vi "Group Terminals.vi"(6 "State":T8={"Worker Library Path"=path "", "Block Label"="", "Types"=[], "Selections"=[], "Icon"={"image type"=0, "image depth"=0, "image"=[], "mask"=[], "colors"=[], "Rectangle"={"left"=0, "top"=0, "right"=0, "bottom"=0}}, "Errors"={"Terminals"=[], "Generate"={"status"=FALSE, "code"=0, "source"=""}, "General"={"status"=FALSE, "code"=0, "source"=""}}, "Calculated Sizes"={"Block Width"=0, "Block Height"=0, "Half Width"=0, "Icon Top"=0, "Icon Bottom"=0, "Label Width"=0, "Half Label"=0, "Label Top"=0, "Text Width"=0, "Half Text"=0, "Text Height"=0, "Label Height"=0, "Expanded Width"=0, "Label Bottom"=0, "Expanded Top"=0, "Expanded Bottom"=0, "Expanded Height"=0, "Min Height"=0, "Max Height"=0}, "Special Terminal Indices"={"Action"=-1, "Init"=-1, "Tag"=-1, "State in"=-1, "State out"=-1, "Error"=-1}, "Terminals"=[]}, 8 "error in (no error)":errorcluster, 11 "Refs In":T15) -> (0 "error out":errorcluster, 2 "Grouped Terms":T1, 3 "Refs":T15)   [LabVIEW 2022 SP3, in "FlexBlocks Support.lvlib"]
uses:
  FlexBlocks Support.lvlib
  SM Refs.ctl
  Flex Block/State.ctl
  Type Descriptor.ctl
  Terminal Direction.ctl
  Value Mode.ctl
  Special Terminal.ctl
  <vilib>/picture/picture.llb/imagedata.ctl
  XNode Errors.ctl
  Calculated Sizes.ctl
  Special Terminal Indices.ctl
  Terminal Status.ctl
  Grouped Terms.ctl
  Terminal Group.ctl
  Terminal State.ctl
  Terminal Draw Style.ctl
  Flex Block/Flex Block.xnode
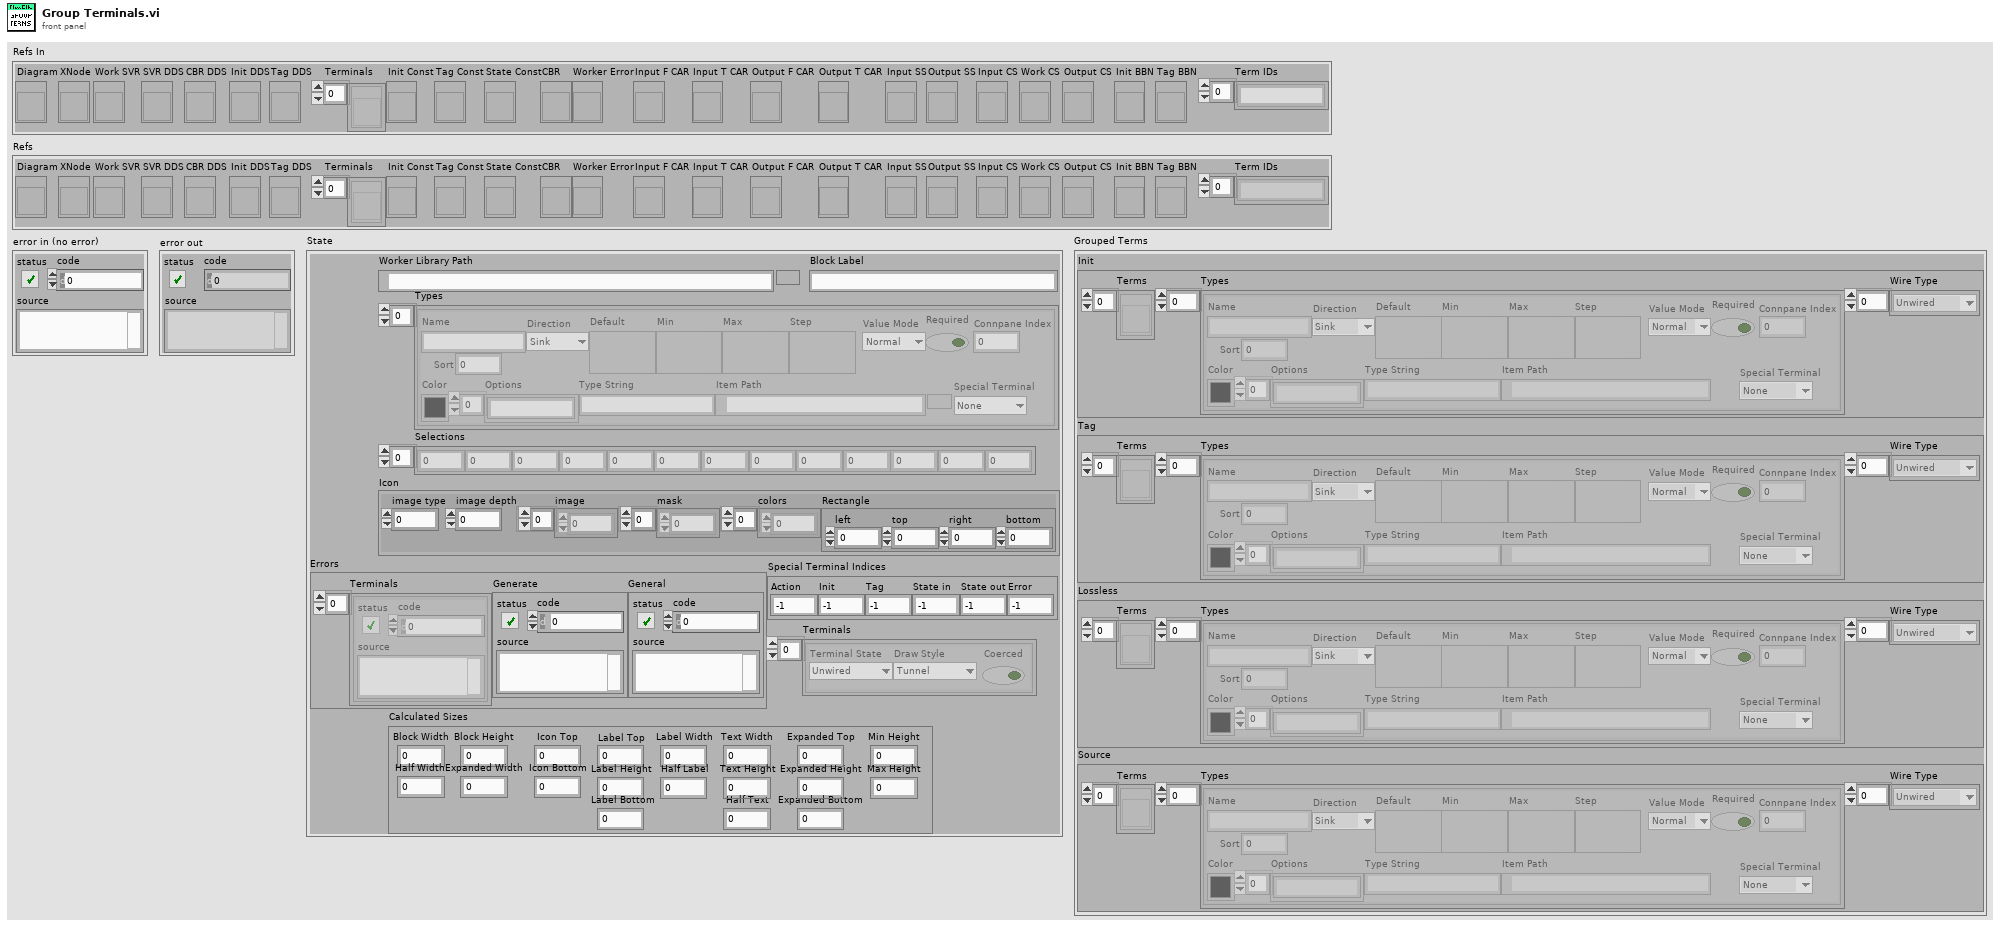
[diagram p1: front panel]
types:
  T1 = typedef "FlexBlocks Support.lvlib/Grouped Terms.ctl" = cluster{"Init":T2, "Tag":T2, "Lossless":T2, "Source":T2}
  T2 = typedef "FlexBlocks Support.lvlib/Terminal Group.ctl" = cluster{"Terms":refnum<vi>[], "Types":T3[], "Wire Type":T7[]}
  T3 = typedef "FlexBlocks Support.lvlib/Type Descriptor.ctl" = cluster{"Name":string, "Direction":T4, "Default":variant, "Min":variant, "Max":variant, "Step":variant, "Value Mode":T5, "Color":u32, "Options":string[], "Type String":string, "Item Path":path, "Required":bool, "Connpane Index":i32, "Special Terminal":T6, "Sort":i32}
  T4 = typedef "FlexBlocks Support.lvlib/Terminal Direction.ctl" = enum16{"Sink", "Source"}
  T5 = typedef "FlexBlocks Support.lvlib/Value Mode.ctl" = enum16{"Normal", "Range", "Select"}
  T6 = typedef "FlexBlocks Support.lvlib/Special Terminal.ctl" = enum16{"None", "Action", "Init", "Tag", "State in", "State out", "Error"}
  T7 = typedef "FlexBlocks Support.lvlib/Terminal State.ctl" = enum16{"Unwired", "BadType", "BadRef", "Channel", "Value", "Control Ref"}
  T8 = typedef "Flex Block.xnode/State.ctl" = cluster{"Worker Library Path":path, "Block Label":string, "Types":T3[], "Selections":i32[], "Icon":T9, "Errors":T10, "Calculated Sizes":T11, "Special Terminal Indices":T12, "Terminals":T13[]}
  T9 = typedef "imagedata.ctl" = cluster{"image type":i32, "image depth":i32, "image":u8[], "mask":u8[], "colors":u32[], "Rectangle":cluster{"left":i16, "top":i16, "right":i16, "bottom":i16}}
  T10 = typedef "FlexBlocks Support.lvlib/XNode Errors.ctl" = cluster{"Terminals":errorcluster[], "Generate":errorcluster, "General":errorcluster}
  T11 = typedef "FlexBlocks Support.lvlib/Calculated Sizes.ctl" = cluster{"Block Width":i32, "Block Height":i32, "Half Width":i32, "Icon Top":i32, "Icon Bottom":i32, "Label Width":i32, "Half Label":i32, "Label Top":i32, "Text Width":i32, "Half Text":i32, "Text Height":i32, "Label Height":i32, "Expanded Width":i32, "Label Bottom":i32, "Expanded Top":i32, "Expanded Bottom":i32, "Expanded Height":i32, "Min Height":i32, "Max Height":i32}
  T12 = typedef "FlexBlocks Support.lvlib/Special Terminal Indices.ctl" = cluster{"Action":i32, "Init":i32, "Tag":i32, "State in":i32, "State out":i32, "Error":i32}
  T13 = typedef "FlexBlocks Support.lvlib/Terminal Status.ctl" = cluster{"Terminal State":T7, "Draw Style":T14, "Coerced":bool}
  T14 = typedef "FlexBlocks Support.lvlib/Terminal Draw Style.ctl" = enum16{"Tunnel", "BadType", "BadRef", "Channel", "Value", "Control Ref"}
  T15 = typedef "FlexBlocks Support.lvlib/SM Refs.ctl" = cluster{"Diagram":refnum<vi>, "XNode":refnum<vi>, "Work SVR":refnum<vi>, "SVR DDS":refnum<vi>, "CBR DDS":refnum<vi>, "Init DDS":refnum<vi>, "Tag DDS":refnum<vi>, "Terminals":refnum<vi>[], "Init Const":refnum<vi>, "Tag Const":refnum<vi>, "State Const":refnum<vi>, "CBR":refnum<vi>, "Worker Error":refnum<vi>, "Input F CAR":refnum<vi>, "Input T CAR":refnum<vi>, "Output F CAR":refnum<vi>, "Output T CAR":refnum<vi>, "Input SS":refnum<vi>, "Output SS":refnum<vi>, "Input CS":refnum<vi>, "Work CS":refnum<vi>, "Output CS":refnum<vi>, "Init BBN":refnum<vi>, "Tag BBN":refnum<vi>, "Term IDs":string[]}
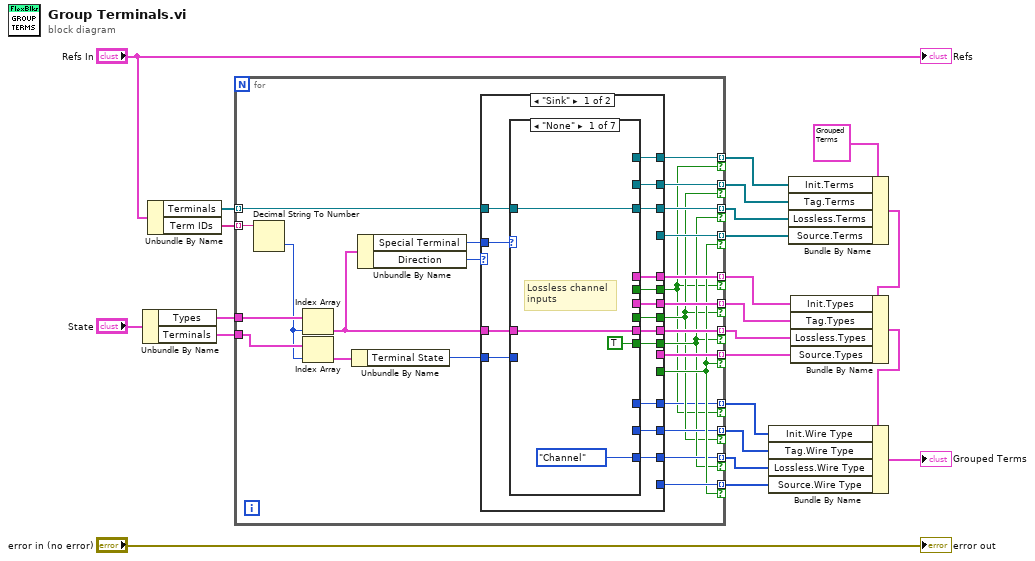
[diagram p0: block diagram]
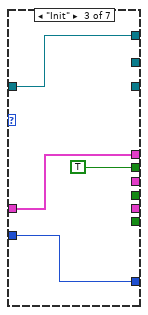
[diagram p3: hidden frame]
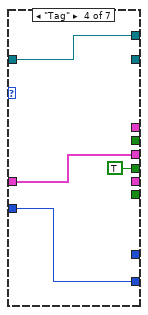
[diagram p4: hidden frame]
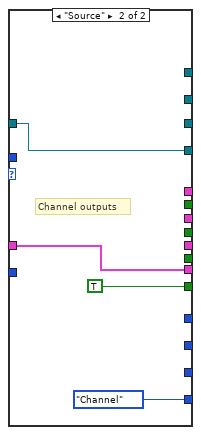
[diagram p8: hidden frame]
diagram:
  n1 = Unbundle By Name("State") -> ("Types"=w22:T3[], "Terminals"=w6:T13[])
  n2 = Unbundle By Name("Refs In") -> ("Terminals"=w21:refnum<vi>[], "Term IDs"=w20:string[])
  n3 = for {
    tunnel: w22 -> [w48]
    tunnel: w21 -> [w45] mode=indexing
    tunnel: w20 -> [w49] mode=indexing
    tunnel: [w43] -> w11 mode=indexing if=w30
    tunnel: [w42] -> w16 mode=indexing if=w30
    tunnel: [w41] -> w9 mode=indexing if=w26
    tunnel: [w40] -> w15 mode=indexing if=w26
    tunnel: [w39] -> w14 mode=indexing if=w24
    tunnel: [w38] -> w8 mode=indexing if=w24
    tunnel: [w37] -> w10 mode=indexing if=w27
    tunnel: [w36] -> w13 mode=indexing if=w27
    tunnel: w6 -> [w35]
    tunnel: [w31] -> w5 mode=indexing if=w30
    tunnel: [w29] -> w3 mode=indexing if=w27
    tunnel: [w28] -> w2 mode=indexing if=w26
    tunnel: [w25] -> w1 mode=indexing if=w24
    n4 = Decimal String To Number(string=w49) -> (number=w34:i32)  [unwired: 2 in, 1 out]
    n5 = Index Array(array=w48, index=w34) -> (element=w44:T3)
    n6 = Index Array(array=w35, index=w34) -> (element=w33:T13)
    n7 = Unbundle By Name(w33) -> ("Terminal State"=w32:T7)
    n8 = Unbundle By Name(w44) -> ("Special Terminal"=w46:T6, "Direction"=w47:T4)
    n9 = case shown="\"Sink\"" w47 {
      tunnel: w46 -> [w65 _]
      tunnel: w45 -> [w63 w79]
      tunnel: w44 -> [w64 w81]
      tunnel: [_ w81] -> w43
      tunnel: [_ w79] -> w42
      tunnel: [_ TRUE] -> w30
      tunnel: [w62 _] -> w41
      tunnel: [w61 _] -> w26
      tunnel: [w60 _] -> w40
      tunnel: [w59 _] -> w39
      tunnel: [w58 _] -> w38
      tunnel: [w57 _] -> w24
      tunnel: [w56 _] -> w37
      tunnel: [w55 _] -> w27
      tunnel: [w54 _] -> w36
      tunnel: w32 -> [w53 _]
      tunnel: [_ Terminal_State."Channel" ("Draw Style")] -> w31
      tunnel: [w52 _] -> w29
      tunnel: [w51 _] -> w28
      tunnel: [w50 _] -> w25
      frame "Sink" {
        n10 = case shown="\"None\"" w65 {
          tunnel: w64 -> [w69 _ w72 w77 _ _ _]
          tunnel: w63 -> [w67 _ w73 w75 _ _ _]
          tunnel: [_ _ _ w77 _ _ _] -> w62
          tunnel: [_ _ _ TRUE _ _ _] -> w61
          tunnel: [_ _ _ w75 _ _ _] -> w60
          tunnel: [_ _ w73 _ _ _ _] -> w59
          tunnel: [_ _ w72 _ _ _ _] -> w58
          tunnel: [_ _ TRUE _ _ _ _] -> w57
          tunnel: [w69 _ _ _ _ _ _] -> w56
          tunnel: [TRUE _ _ _ _ _ _] -> w55
          tunnel: [w67 _ _ _ _ _ _] -> w54
          tunnel: w53 -> [_ _ w70 w74 _ _ _]
          tunnel: [Terminal_State."Channel" ("Draw Style") _ _ _ _ _ _] -> w52
          tunnel: [_ _ _ w74 _ _ _] -> w51
          tunnel: [_ _ w70 _ _ _ _] -> w50
          frame "None" {
            # "Lossless channel inputs"
          }
          frame "Action" {
          }
          frame "Init" {
          }
          frame "Tag" {
          }
          frame "State in" {
          }
          frame "State out" {
          }
          frame "Error" {
          }
        }
      }
      frame "Source" {
        # "Channel outputs"
      }
    }
  }
  n11 = Bundle By Name(cluster=T1 {"Init"={"Terms"=[], "Types"=[], "Wire Type"=[]}, "Tag"={"Terms"=[], "Types"=[], "Wire Type"=[]}, "Lossless"={"Terms"=[], "Types"=[], "Wire Type"=[]}, "Source"={"Terms"=[], "Types"=[], "Wire Type"=[]}} ("Grouped Terms"), "Init.Terms"=w14, "Tag.Terms"=w15, "Lossless.Terms"=w13, "Source.Terms"=w16) -> (w12:T1)
  n12 = Bundle By Name(cluster=w12, "Init.Types"=w8, "Tag.Types"=w9, "Lossless.Types"=w10, "Source.Types"=w11) -> (w7:T1)
  n13 = Bundle By Name(cluster=w7, "Init.Wire Type"=w1, "Tag.Wire Type"=w2, "Lossless.Wire Type"=w3, "Source.Wire Type"=w5) -> (→"Grouped Terms":T1)
  "Refs" <- "Refs In"
  "error out" <- "error in (no error)"
